vi "Initialcharge.vi"(5 "Path":path, 6 "Resistance Setpoint (0 Ohms)":dbl format="%#.6g", 7 "VISA resource name":refnum<visa-resource-name>, 8 "Power Setpoint (0 W)":dbl format="%#.6g", 9 "Current Setpoint (0 A)":dbl format="%#.6g", 10 "Voltage Setpoint (0 V)":dbl format="%#.6g", 11 "Battery Detect Voltage (0V)":dbl format="%#.6g") -> ()   [LabVIEW 2020]
uses:
  65859b5f-dbaa-4545-a529-31588f6a908f.vi
  59f29fdb-980d-4932-87e1-4cec12b2c3d3.vi
  <instrlib>/NH Research Regenerative Test Series/Public/Data/Read (Ave Current).vi
  <instrlib>/NH Research Regenerative Test Series/Public/Data/Low Level/Fetch (Ave Voltage).vi
  <instrlib>/NH Research Regenerative Test Series/Public/Data/Low Level/Fetch (Ave True Power).vi
  <instrlib>/NH Research Regenerative Test Series/NH Research Regenerative Test Series.lvlib
panel:
  out "Ave Current (A)":dbl
  out "Ave Voltage (V)":dbl
  out "Ave True Power (W)":dbl
  out "Status Byte Register":T1
  in  "Logical Instrument Number":u32=1
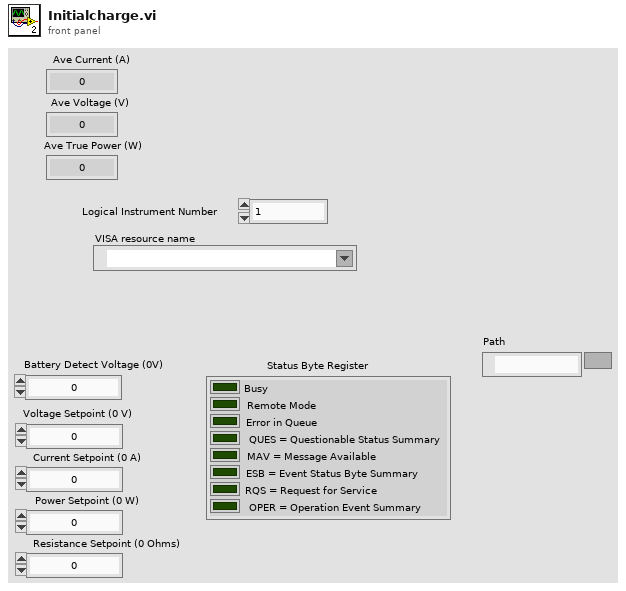
[diagram p1: front panel]
types:
  T1 = cluster{"Busy":bool, "Remote Mode":bool, "Error in Queue":bool, "QUES = Questionable Status Summary":bool, "MAV = Message Available":bool, "ESB = Event Status Byte Summary":bool, "RQS = Request for Service":bool, "OPER = Operation Event Summary":bool}
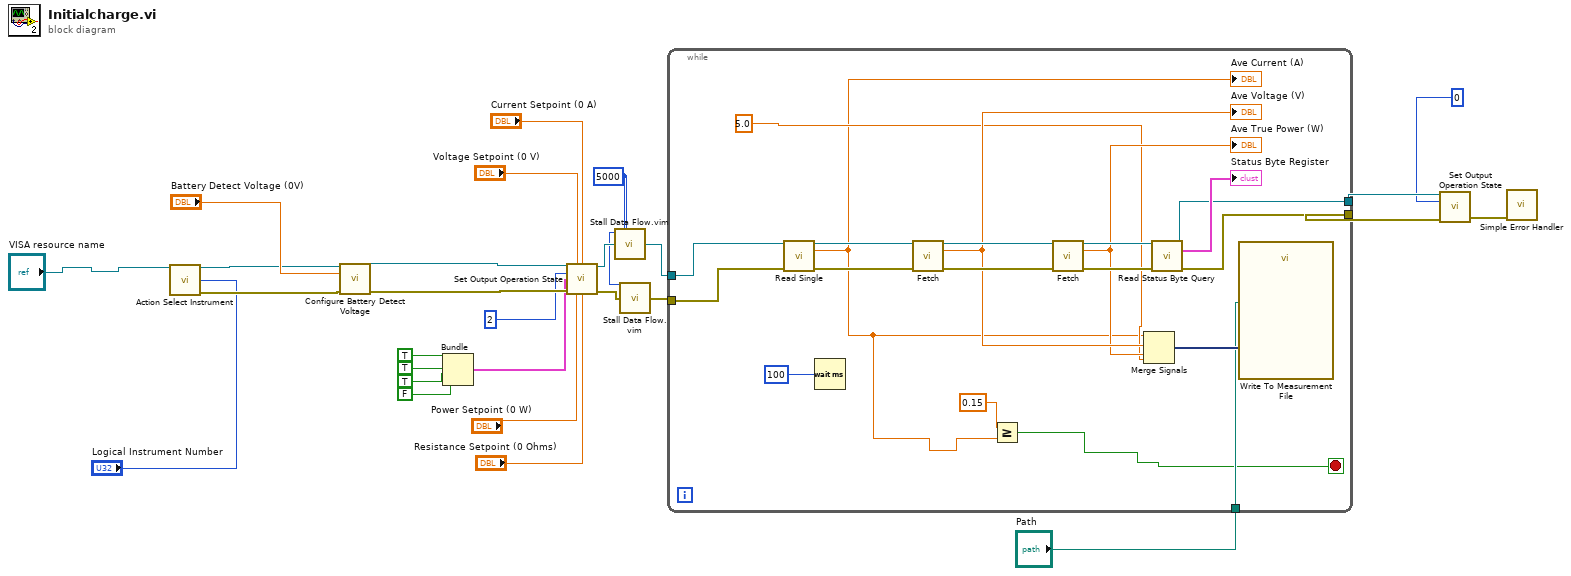
[diagram p0: block diagram]
diagram:
  w1 = 5000
  n1 = call <instrlib>:"Action Select Instrument.vi"("VISA resource name"="VISA resource name", "Logical Instrument Number"="Logical Instrument Number") -> ("VISA resource name out"=w22:refnum<visa-resource-name>, "error out"=w21:errorcluster)  [unwired: 12 in]
  n2 = call <vilib>:"Configure Battery Detect Voltage.vi"("VISA resource name"=w22, "Battery Detect Voltage (0V)"="Battery Detect Voltage (0V)", "error in (no error)"=w21) -> ("VISA resource name out"=w20:refnum<visa-resource-name>, "error out"=w19:errorcluster)  [unwired: 11 in]
  n3 = Bundle(TRUE, TRUE, TRUE, FALSE) -> (w8:cluster{bool, bool, bool, bool})  [unwired: 1 in]
  n4 = call <vilib>:"Set Output Operation State.vi"("VISA resource name"=w20, "Voltage Setpoint (0 V)"="Voltage Setpoint (0 V)", "Current Setpoint (0 A)"="Current Setpoint (0 A)", "Mode (0: Off)"=2, "Enable"=w8, "error in (no error)"=w19, "Power Setpoint (0 W)"="Power Setpoint (0 W)", "Resistance Setpoint (0 Ohms)"="Resistance Setpoint (0 Ohms)") -> ("VISA resource name out"=w5:refnum<visa-resource-name>, "error out"=w3:errorcluster)  [unwired: 6 in]
  n5 = call "Stall Data Flow.vim"("value in"=w5, "milliseconds to wait"=w1) -> ("value out"=w4:refnum<visa-resource-name>)  [unwired: 1 out]
  n6 = call "Stall Data Flow.vim"("value in"=w3, "milliseconds to wait"=w1) -> ("value out"=w2:errorcluster)  [unwired: 1 out]
  n7 = while {
    tunnel: w4 -> [w40]
    tunnel: w2 -> [w39]
    tunnel: [w37] -> w18
    tunnel: [w36] -> w17
    tunnel: "Path" -> [w32]
    stop <- w29 stop-if-true
    n8 = call-poly <instrlib>:"Read Single.vi"("VISA resource name"=w40, "error in (no error)"=w39) -> ("VISA resource name out"=w45:refnum<visa-resource-name>, "Ave Current (A)"=w28:dbl, "error out"=w46:errorcluster)  [unwired: 11 in]
    "Ave Current (A)" <- w28
    n9 = Wait (ms)(milliseconds to wait=100) -> ()  [unwired: 1 out]
    n10 = call-poly <instrlib>:"Fetch.vi"("VISA resource name"=w45, "error in (no error)"=w46) -> ("VISA resource name out"=w44:refnum<visa-resource-name>, "Ave Voltage (V)"=w35:dbl, "error out"=w43:errorcluster)  [unwired: 11 in]
    "Ave Voltage (V)" <- w35
    n11 = Greater Or Equal?(x=0.15, y=w28) -> (x >= y?=w29:bool)
    n12 = call-poly <instrlib>:"Fetch.vi"("VISA resource name"=w44, "error in (no error)"=w43) -> ("VISA resource name out"=w42:refnum<visa-resource-name>, "Ave True Power (W)"=w34:dbl, "error out"=w41:errorcluster)  [unwired: 11 in]
    "Ave True Power (W)" <- w34
    n13 = Merge Signals "Merge Signals"(w28, w35, w34, 5.0) -> (w47:dynamicdata)
    n14 = call <instrlib>:"Read Status Byte Query.vi"("VISA resource name"=w42, "error in (no error)"=w41) -> ("VISA resource name out"=w37:refnum<visa-resource-name>, "Status Byte Register"=→"Status Byte Register":T1, "error out"=w36:errorcluster)  [unwired: 11 in]
    n15 = call "Write To Measurement File"("Signals"=w47, "Filename"=w32) -> ()  [unwired: 15 in, 3 out]
  }
  n16 = call <vilib>:"Set Output Operation State.vi"("VISA resource name"=w18, "Mode (0: Off)"=0, "error in (no error)"=w17) -> ("error out"=w7:errorcluster)  [unwired: 11 in, 1 out]
  n17 = call <vilib>:"Simple Error Handler.vi"("error in (no error)"=w7) -> ()  [unwired: 4 in, 5 out]
